vi "do show conditional terminal.vi"(8 "error in (no error)":errorcluster, 10 "show_conditional_terminal Argument":T3, 11 "Data Cluster in":T1) -> (0 "error out":errorcluster, 2 "show_conditional_terminal (Reply Payload)":T2, 3 "Data Cluster out":T1)   [LabVIEW 2025, in "Scripting Server.lvlib"]
uses:
  Scripting Server.lvlib
  show_conditional_terminal (Reply Payload)--cluster.ctl
  Module Data--cluster.ctl
  show_conditional_terminal Argument--cluster.ctl
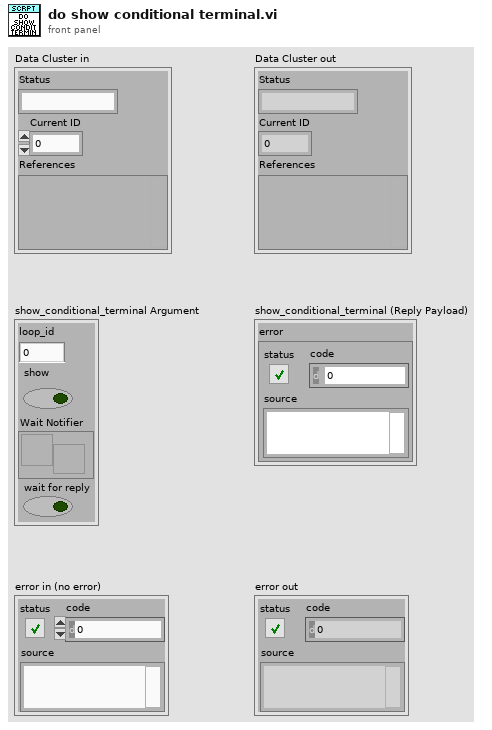
[diagram p1: front panel]
types:
  T1 = typedef "Scripting Server.lvlib/Module Data--cluster.ctl" = cluster{"Status":string, "Current ID":i32, "References":variant}
  T2 = typedef "Scripting Server.lvlib/show_conditional_terminal (Reply Payload)--cluster.ctl" = cluster{"error":errorcluster}
  T3 = typedef "Scripting Server.lvlib/show_conditional_terminal Argument--cluster.ctl" = cluster{"loop_id":i32, "show":bool, "Wait Notifier":refnum<notifier>, "wait for reply":bool}
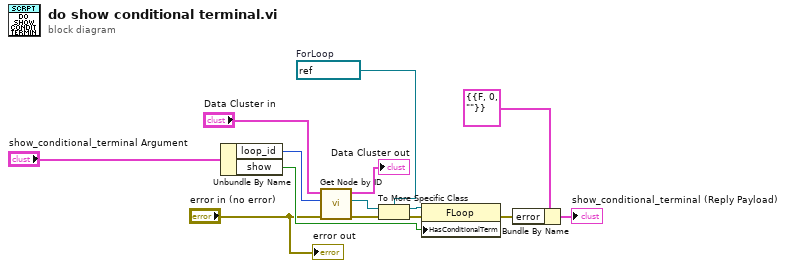
[diagram p0: block diagram]
diagram:
  w6 = refnum<vi> refnum  # ForLoop
  n1 = Unbundle By Name("show_conditional_terminal Argument") -> ("loop_id"=w9:i32, "show"=w3:bool)
  n2 = call "Get Node by ID.vi"("error in (no error)"="error in (no error)", "ID"=w9, "Data Cluster in"="Data Cluster in") -> ("error out"=w11:errorcluster, "specific class reference"=w7:refnum<vi>, "Data Cluster out"=→"Data Cluster out":T1)  [unwired: 6 in]
  n3 = To More Specific Class(target class=w6, reference=w7, error in=w11) -> (specific class reference=w5:refnum<vi>, error out=w8:errorcluster)
  n4 = property class="FLoop"(reference=w5, error in=w8, "HasConditionalTerm"=w3) -> (error out=w2:errorcluster)  [unwired: 1 out]
  n5 = Bundle By Name(cluster=T2 {"error"={"status"=FALSE, "code"=0, "source"=""}} ("show_conditional_terminal (Reply Payload)"), "error"=w2) -> (→"show_conditional_terminal (Reply Payload)":T2)
  "error out" <- "error in (no error)"
